vi "AO Check For Empty Channels.vi"(1 "AO Configuration In":T1(array[cluster])=[{"Output physical channels"="PXI1Slot2/ao0:1", "AO. Max"=0.1, "AO.Min"=-0.1}, {"Output physical channels"="PXI1Slot3/ao0:1", "AO. Max"=0.1, "AO.Min"=-0.1}, {"Output physical channels"="PXI1Slot6/ao0:1", "AO. Max"=0.0, "AO.Min"=0.0}]) -> (0 "AO Configuration Out":T1(array[cluster]))   [LabVIEW 2013, in "Lock-In Variable Channels_2.lvclass"]
uses:
  Lock-In Variable Channels_2.lvclass
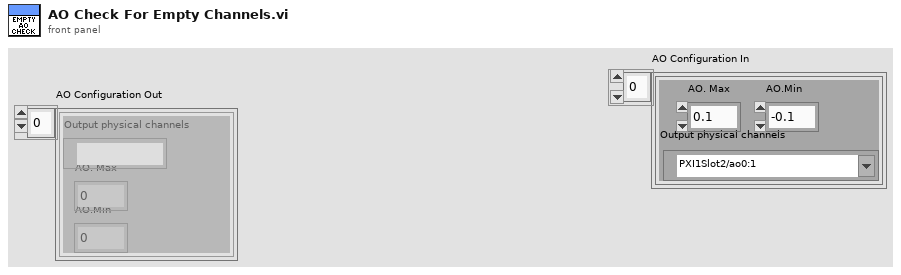
[diagram p1: front panel]
types:
  T1 = cluster{"Output physical channels":tag, "AO. Max":dbl, "AO.Min":dbl}[]
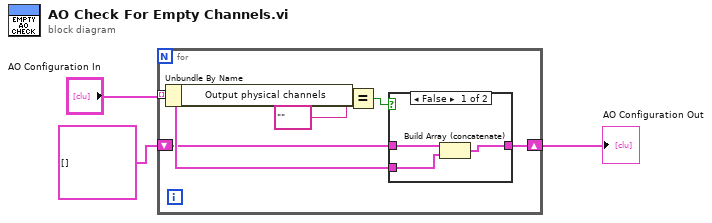
[diagram p0: block diagram]
diagram:
  n1 = for {
    tunnel: "AO Configuration In" -> [w6] mode=indexing
    shift-right: [w4] -> w1
    shift-left: T1 [] ("AO Configuration 2") -> [w5]
    n2 = Unbundle By Name(w6) -> ("Output physical channels"=w8:tag)
    n3 = Equal?(x=w8, y=tag "" ("Empty physical channels")) -> (x = y?=w9:bool)
    n4 = case shown="False" w9 {
      tunnel: w6 -> [w11 _]
      tunnel: w5 -> [w12 w13]
      tunnel: [w10 w13] -> w4
      frame False {
        n5 = Build Array (concatenate)(w12, w11) -> (w10:T1)
      }
      frame True {
      }
    }
  }
  "AO Configuration Out" <- w1
